vi "tcpExampleServer.vi"() -> ()   [LabVIEW 2014]
uses:
  typedefs/clientStatus.ctl
  typedefs/clientConfiguration.ctl
panel:
  out "server status":T1
  out "receive client->server":string
  in  "transmit server->client":string
  in  "stop":bool
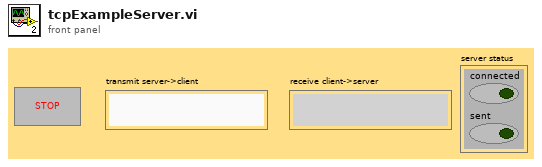
[diagram p1: front panel]
types:
  T1 = typedef "clientStatus.ctl" = cluster{"connected":bool, "sent":bool}
  T2 = typedef "clientConfiguration.ctl" = cluster{"client ID":string, "remote host":string, "local port":u16, "remote port":u16}
  T3 = typedef "QueueCluster.ctl" = cluster{"status":cluster{"queue":refnum<queue>, "error out":errorcluster}, "receive":cluster{"queue":refnum<queue>, "error out":errorcluster}, "transmit":cluster{"queue":refnum<queue>, "error out":errorcluster}, "shutdown":cluster{"queue":refnum<queue>, "error out":errorcluster}, "semaphore":T4}
  T4 = typedef "Semaphore RefNum" = refnum<k1>
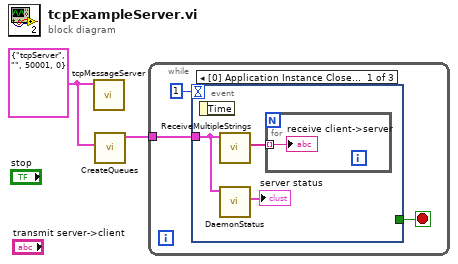
[diagram p0: block diagram]
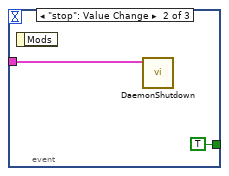
[diagram p2: hidden frame]
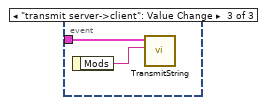
[diagram p3: hidden frame]
diagram:
  w2 = T2 {"client ID"="tcpServer", "remote host"="", "local port"=50001, "remote port"=0} ("client configuration")
  n1 = call "tcpMessageServer.vi"("server configuration"=w2) -> ()  [unwired: 10 in, 1 out]
  n2 = call "CreateQueues.vi"("client configuration"=w2) -> ("output cluster"=w1:T3)  [unwired: 10 in]
  n3 = while {
    tunnel: w1 -> [w4]
    stop <- w5 stop-if-true
    n4 = event shown="[0] Application Instance Close?" {
      selector: _ -> [_ _ _]
      dyn-events: _ -> [_ _ _]
      timeout: 1 -> [_ _ _]
      tunnel: [_ TRUE _] -> w5
      tunnel: w4 -> [w8 w10 w13]
      event Timeout {
        n5 = event-data() -> ()  [unwired: 1 in, 1 out]
        n6 = call "ReceiveMultipleStrings.vi"("queue cluster"=w8) -> ("received strings"=w6:string[])  [unwired: 7 in, 3 out]
        n7 = call "DaemonStatus.vi"("queue cluster"=w8) -> ("status"=→"server status":T1)  [unwired: 8 in, 2 out]
        n8 = for {
          tunnel: w6 -> [w9] mode=indexing
          "receive client->server" <- w9
        }
      }
      event "stop": Value Change {
        n9 = event-data() -> ()  [unwired: 1 in, 1 out]
        n10 = call "DaemonShutdown.vi"("queue cluster"=w10) -> ()  [unwired: 9 in, 2 out]
      }
      event "transmit server->client": Value Change {
        n11 = event-data() -> ("Mods"=w12:string)  [unwired: 1 in]
        n12 = call "TransmitString.vi"("string to transmit"=w12, "queue cluster"=w13) -> ()  [unwired: 8 in, 2 out]
      }
    }
  }
